vi "Error Offset (Configuration).vi"() -> (3 "error code offset":i32)   [LabVIEW 2017, in "DSF Core.lvlib"]
uses:
  DSF Core.lvlib
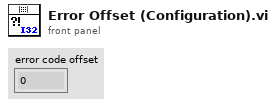
[diagram p1: front panel]
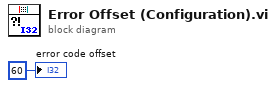
[diagram p0: block diagram]
diagram:
  "error code offset" <- 60 ("base error code")
